vi "Preset_to_Array.vi"(10 "Preset Name":string) -> (1 "Column Headers":string[](array[string])=["Device Name", "Device Variable", "Preset Value"], 3 "Preset Table":string[][](array[string]))   [LabVIEW 2020]
uses:
  Shared/MySQL/Preset Query Enum.ctl
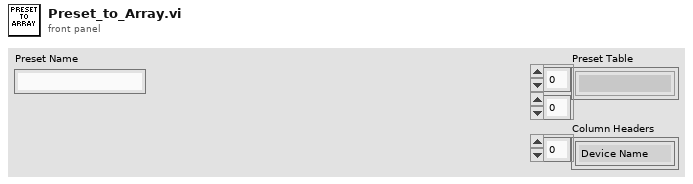
[diagram p1: front panel]
types:
  T1 = typedef "Preset Query Enum.ctl" = enum16{"Get Locations", "Get all IPs and MACs", "Get classes", "Get expt variables to set at scanstart for particular device", "Get expt devices and variables with start values", "Get expt devices and variables (with data to get)", "Get expt devices with data to get", "Get Expt devices and GUIs", "Get all devices basic properties", "Get Virtual Devices Core Info", "Get Expt names", "Get experiment basic properties", "Get experiment alarm variables", "Get MC Ports", "Get device network comm port", "Get devicetype lvclass path", "Get basic device properties", "Get Init Order", "Get all setable variables of a device", "Get device variable aliases", "Get force values of all settable variables", "Get all variables of a devicetype", "Get all variables of a device", "Get plotter details", "Get Saved Scans", "Get Scan Info", "GetGeneralGUIs", "Get expt for plotter", "Get plotter IDs from expt", "Get all devices", "Get all Virtual Devices", "Get all aliases", "Get variable and device info for Virtual Device", "GetItemLocatorIP", "Get IPs for GUIs", "Get DeviceType from Device", "GetLocalPortRange", "GetDevicePresetVariables", "Get Device Configuration", "GetAllPresetNames", "GetAllConfigurationNames", "GetPresetDeviceNames", "GetDeviceAliases", "GetDevicesOfClass"}
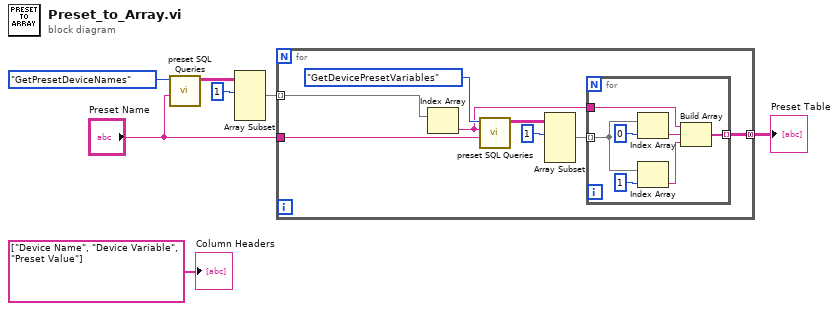
[diagram p0: block diagram]
diagram:
  n1 = call "preset SQL Queries.vi"("Expt name / MCIP/ Variable/Preset Name"="Preset Name", "Preset Query"=Preset_Query_Enum."GetPresetDeviceNames") -> ("data"=w6:string[][])  [unwired: 7 in, 2 out]
  n2 = Array Subset(array=w6, index (row)=1 ("index")) -> (w4:string[][])  [unwired: 3 in]
  n3 = for {
    tunnel: w4 -> [w11] mode=indexing
    tunnel: "Preset Name" -> [w12]
    tunnel: [w8] -> w3 mode=concatenating
    n4 = Index Array(array=w11) -> (element=w9:string)  [unwired: 1 in]
    n5 = call "preset SQL Queries.vi"("Expt name / MCIP/ Variable/Preset Name"=w12, "Device/Devicetype name\n/Plotter.id/ScanName#"=w9, "Preset Query"=Preset_Query_Enum."GetDevicePresetVariables") -> ("data"=w14:string[][])  [unwired: 6 in, 2 out]
    n6 = Array Subset(array=w14, index (row)=1 ("index")) -> (w10:string[][])  [unwired: 3 in]
    n7 = for {
      tunnel: w10 -> [w20] mode=indexing
      tunnel: [w19] -> w8 mode=indexing
      tunnel: w9 -> [w16]
      n8 = Index Array(array=w20, index=0 ("index (row)")) -> (element=w18:string)
      n9 = Index Array(array=w20, index=1 ("disabled index (col)")) -> (element=w17:string)
      n10 = Build Array(w16, w18, w17) -> (w19:string[])
    }
  }
  "Preset Table" <- w3
  "Column Headers" <- string[] ["Device Name", "Device Variable", "Preset Value"] ("Column Headers")
